vi "Actor Core.vi"(8 "error in":errorcluster, 11 "Panel Form Controller in":refnum<class "Panel Form Controller.lvclass">) -> (0 "error out":errorcluster, 3 "Actor out":refnum<class "Actor.lvclass">)   [LabVIEW 2020, in "Panel Form Controller.lvlib" / "Panel Form Controller.lvclass"]
doc: "The user interface for this panel.\n\n----\nPlease see the following web address for additional documentation and tutorial information:\nhttp://www.mooregoodideas.com/mgi-panel-manager/\n\nAuthor: Derek Trepanier\n\nCopyright (c) 2018, Moore Good Ideas, Inc.\n\nAll rights reserved.\n\nRedistribution and use in source and binary forms, with or without modification, are permitted provided that the following conditions are met:\n\n * Redistributions of source code must retain the above copyright notice, this list of conditions and the following disclaimer.\n * Redistributions in binary form must reproduce the above copyright notice, this list of conditions and the following disclaimer in the documentation and/or other materials provided with the distribution.\n * Neither the name of Moore Good Ideas, Inc. nor the names of its contributors may be used to endorse or promote products derived from this software without specific prior written permission.\n\nTHIS SOFTWARE IS PROVIDED BY THE COPYRIGHT HOLDERS AND CONTRIBUTORS \"AS IS\" AND ANY EXPRESS OR IMPLIED WARRANTIES, INCLUDING, BUT NOT LIMITED TO, THE IMPLIED WARRANTIES OF MERCHANTABILITY AND FITNESS FOR A PARTICULAR PURPOSE ARE DISCLAIMED. IN NO EVENT SHALL THE COPYRIGHT OWNER OR CONTRIBUTORS BE LIABLE FOR ANY DIRECT, INDIRECT, INCIDENTAL, SPECIAL, EXEMPLARY, OR CONSEQUENTIAL DAMAGES (INCLUDING, BUT NOT LIMITED TO, PROCUREMENT OF SUBSTITUTE GOODS OR SERVICES; LOSS OF USE, DATA, OR PROFITS; OR BUSINESS INTERRUPTION) HOWEVER CAUSED AND ON ANY THEORY OF LIABILITY, WHETHER IN CONTRACT, STRICT LIABILITY, OR TORT (INCLUDING NEGLIGENCE OR OTHERWISE) ARISING IN ANY WAY OUT OF THE USE OF THIS SOFTWARE, EVEN IF ADVISED OF THE POSSIBILITY OF SUCH DAMAGE."
uses:
  Panel Form Controller.lvclass
  C:/Program Files (x86)/National Instruments/LabVIEW 2020/vi.lib/MGI/Panel Manager/Panel Actor/Panel Actor/Panel Actor.lvclass
  C:/Program Files (x86)/National Instruments/LabVIEW 2020/vi.lib/ActorFramework/Actor/Actor.lvclass
  <vilib>/ActorFramework/Actor/Actor.lvclass
  <vilib>/MGI/Panel Manager/Panel/Panel Helper/Panel Events.ctl
  <vilib>/MGI/Panel Manager/Panel/Panel Helper/Events.ctl
  Database OOP/Open Form Button/Open Form Button Class/Open Form.lvclass
  <vilib>/ActorFramework/Actor/Actor.lvclass/Actor.ctl
  Panel Form Controller.lvclass/Panel Form Controller.ctl
  Database OOP/Open Form Button/Open Form Button Class/Open Form.lvclass/Open Form.ctl
  Form Model Messages Messages/Open Form Msg/Open Form Msg.lvclass/Open Form Msg.ctl
  <vilib>/ActorFramework/Message Enqueuer/Message Enqueuer.lvclass/Message Enqueuer.ctl
  <vilib>/ActorFramework/Message Enqueuer/Enqueue.vi
  Form Model Messages Messages/Open Form Msg/Open Form Msg.lvclass
  C:/Program Files (x86)/National Instruments/LabVIEW 2020/vi.lib/ActorFramework/Message/Message.lvclass
  <vilib>/ActorFramework/Stop Msg/Stop Msg.lvclass
  <vilib>/ActorFramework/Message Priority Queue/Priority Enqueue.vi
  <vilib>/MGI/Panel Manager/Panel Actor/Panel Actor/Panel Actor.lvclass
  <vilib>/MGI/Panel Manager/Panel/Panel Helper/Panel Helper.lvclass
types:
  T1 = cluster{"Pnl Actor":refnum<event-registration>, "Child Pnl":refnum<event-registration>, "Child Fields":refnum<event-registration>, "Child Buttons":refnum<event-registration>}
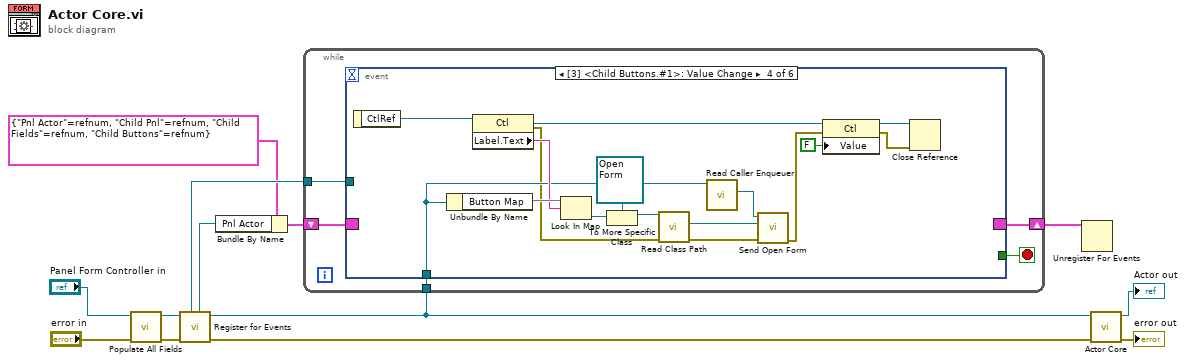
[diagram p0: block diagram]
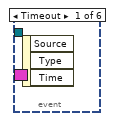
[diagram p2: hidden frame]
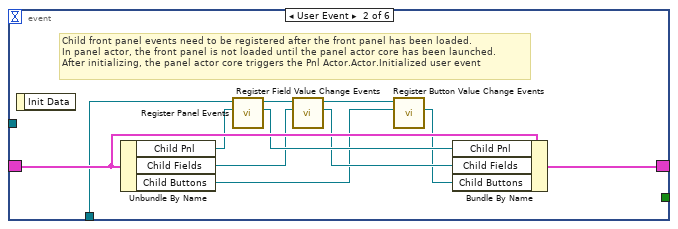
[diagram p3: hidden frame]
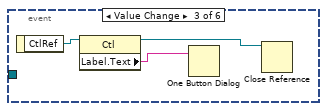
[diagram p4: hidden frame]
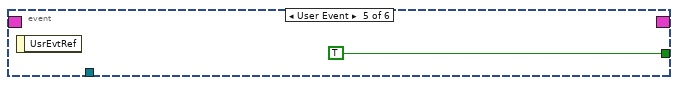
[diagram p5: hidden frame]
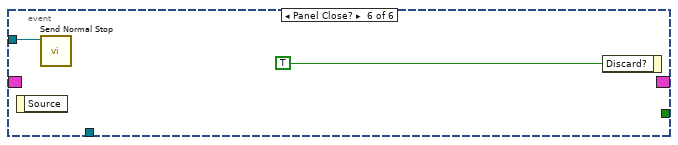
[diagram p6: hidden frame]
diagram:
  n1 = call "Populate All Fields.vi"("error in (no error)"="error in", "Panel Form Controller in"="Panel Form Controller in") -> ("error out"=w1:errorcluster, "Panel Form Controller out"=w3:refnum<class "Panel Form Controller.lvclass">)  [unwired: 8 in]
  n2 = call <vilib>:"Register for Events.vi"("Error In"=w1, "Panel Actor in"=w3) -> ("Error Out"=w6:errorcluster, "Panel Actor out"=w5:refnum<class "Panel Form Controller.lvclass">, "Pnl Actor"=w7:refnum<event-registration>, "Self Enqueuer"=w10:refnum<class "Message Enqueuer.lvclass">)  [unwired: 6 in]
  n3 = Bundle By Name(cluster=T1 {"Pnl Actor"=refnum, "Child Pnl"=refnum, "Child Fields"=refnum, "Child Buttons"=refnum}, "Pnl Actor"=w7) -> (w8:T1)
  n4 = while {
    tunnel: w10 -> [w18]
    tunnel: w5 -> [w14]
    shift-right: [w16] -> w11
    shift-left: w8 -> [w15]
    stop <- w17 stop-if-true
    n5 = event shown="[3] <Child Buttons.#1>: Value Change" {
      selector: w15 -> [_ w29 _ _ _ _]
      dyn-events: [_ w28 _ _ _ _] -> w16
      timeout: _ -> [_ _ _ _ _ _]
      tunnel: w18 -> [_ _ _ _ _ w51]
      tunnel: [_ _ _ _ TRUE _] -> w17
      tunnel: w14 -> [_ w22 _ w41 _ _]
      event Timeout {
        n6 = event-data() -> ()  [unwired: 1 in, 3 out]
      }
      event User Event {
        # "Child front panel events need to be registered after the front panel has been loaded.\nIn panel actor, the front panel is not loaded until the panel actor core has been launched.\nAfter initializing, the panel actor core triggers the Pnl Actor.Actor.Initialized user event"
        n7 = event-data() -> ()  [unwired: 1 in, 1 out]
        n8 = Unbundle By Name(w29) -> ("Child Pnl"=w27:refnum<event-registration>, "Child Fields"=w25:refnum<event-registration>, "Child Buttons"=w20:refnum<event-registration>)
        n9 = call "Register Panel Events.vi"("Event Refnum In"=w27, "Panel Form Controller in"=w22) -> ("Event Refnum Out"=w26:refnum<event-registration>, "Panel Form Controller out"=w23:refnum<class "Panel Form Controller.lvclass">)  [unwired: 7 in, 1 out]
        n10 = call "Register Field Value Change Events.vi"("Field Event Refnum In"=w25, "Panel Form Controller in"=w23) -> ("Field Event Refnum Out"=w24:refnum<event-registration>, "Panel Form Controller out"=w21:refnum<class "Panel Form Controller.lvclass">)  [unwired: 7 in, 1 out]
        n11 = call "Register Button Value Change Events.vi"("Button Event Refnum In"=w20, "Panel Form Controller in"=w21) -> ("Button Event Refnum Out"=w19:refnum<event-registration>)  [unwired: 7 in, 2 out]
        n12 = Bundle By Name(cluster=w29, "Child Pnl"=w26, "Child Fields"=w24, "Child Buttons"=w19) -> (w28:T1)
      }
      event Value Change {
        n13 = event-data() -> ("CtlRef"=w32:refnum<vi>)  [unwired: 1 in]
        n14 = property class="Ctl"(reference=w32) -> (reference out=w30:refnum<vi>, "Label.Text"=w31:string)  [unwired: 1 in, 1 out]
        n15 = One Button Dialog(message=w31) -> ()  [unwired: 1 in, 1 out]
        n16 = Close Reference(reference=w30) -> ()  [unwired: 1 in, 1 out]
      }
      event Value Change {
        n17 = event-data() -> ("CtlRef"=w48:refnum<vi>)  [unwired: 1 in]
        n18 = Unbundle By Name(w41) -> ("Button Map"=w47:map{string, refnum<class "Button.lvclass">})
        n19 = property class="Ctl"(reference=w48) -> (reference out=w39:refnum<vi>, error out=w36:errorcluster, "Label.Text"=w46:string)  [unwired: 1 in]
        n20 = Look In Map(map=w47, key=w46) -> (value=w45:refnum<class "Button.lvclass">)  [unwired: 1 in, 1 out]
        n21 = To More Specific Class(target class=refnum<class "Open Form.lvclass"> refnum ("Open Form Button.lvlib:Open Form.lvclass"), reference=w45) -> (specific class reference=w43:refnum<class "Open Form.lvclass">)  [unwired: 1 in, 1 out]
        n22 = call "Read Class Path.vi"("error in (no error)"=w36, "Open Form in"=w43) -> ("error out"=w33:errorcluster, "Class Path"=w42:path)  [unwired: 7 in, 1 out]
        n23 = call <vilib>:"Read Caller Enqueuer.vi"("Actor"=w41) -> ("Caller Enqueuer"=w40:refnum<class "Message Enqueuer.lvclass">)  [unwired: 10 in]
        n24 = call "Send Open Form.vi"("error in (no error)"=w33, "Form path"=w42, "Message Enqueuer"=w40) -> ("error out"=w35:errorcluster)  [unwired: 7 in, 1 out]
        n25 = property class="Ctl"(reference=w39, error in=w35, "Value"=FALSE) -> (reference out=w37:refnum<vi>, error out=w34:errorcluster)
        n26 = Close Reference(reference=w37, error in (no error)=w34) -> ()  [unwired: 1 out]
      }
      event User Event {
        n27 = event-data() -> ()  [unwired: 1 in, 1 out]
      }
      event Panel Close? {
        n28 = event-data() -> ()  [unwired: 1 in, 1 out]
        n29 = call <vilib>:"Send Normal Stop.vi"("Message Enqueuer"=w51) -> ()  [unwired: 10 in, 1 out]
        n30 = event-data("Discard?"=TRUE) -> ()  [unwired: 1 in, 1 out]
      }
    }
  }
  n31 = Unregister For Events(event registration refnum=w11) -> ()  [unwired: 1 in, 1 out]
  n32 = call-parent "Actor Core.vi"("error in"=w6, "Panel Actor in"=w5) -> ("error out"=→"error out":errorcluster, "Actor out"=→"Actor out":refnum<class "Actor.lvclass">)  [unwired: 8 in]
